vi "Shooter_Globals.vi"() -> ()   [LabVIEW 2020]
uses:
  Shooter_Cluster.ctl
  Shooter_Control_States.ctl
panel:
  in  "Shooter_Determiner_Set_Ref":string="Shooter_Determiner_Set_Ref"
  in  "Shooter_Determiner_Notifier":refnum<notifier>
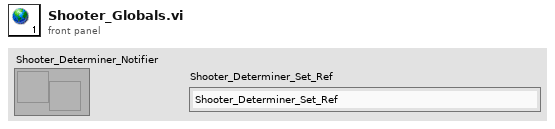
[diagram p1: front panel]
diagram:
